vi "Build Chart.vi"(10 "Translation":dbl[](array[numeric]), 11 "angles (deg)":cluster{"yaw":dbl, "pitch":dbl, "roll":dbl}) -> (3 "chart data":T1)   [LabVIEW 2023]
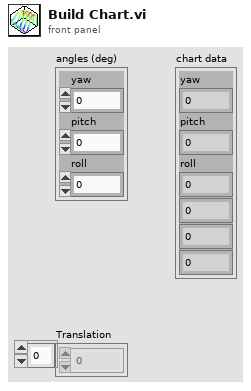
[diagram p1: front panel]
types:
  T1 = cluster{"yaw":dbl, "pitch":dbl, "roll":dbl, dbl, dbl, dbl}
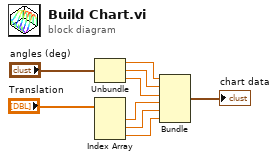
[diagram p0: block diagram]
diagram:
  n1 = Unbundle("angles (deg)") -> ("yaw"=w1:dbl, "pitch"=w2:dbl, "roll"=w3:dbl)
  n2 = Index Array(array="Translation") -> (element #1=w5:dbl, element #2=w6:dbl, element #3=w7:dbl)  [unwired: 3 in]
  n3 = Bundle("yaw"=w1, "pitch"=w2, "roll"=w3, w5, w6, w7) -> (→"chart data":T1)  [unwired: 1 in]
